vi "Finish.vi"(8 "error in (no error)":errorcluster, 11 "System Actor in":refnum<class "System Actor.lvclass">) -> (0 "error out":errorcluster, 3 "System Actor out":refnum<class "System Actor.lvclass">)   [LabVIEW 2014, in "Robot Actor Framework.lvlib" / "System Actor.lvlib" / "System Actor.lvclass"]
uses:
  System Actor.lvclass
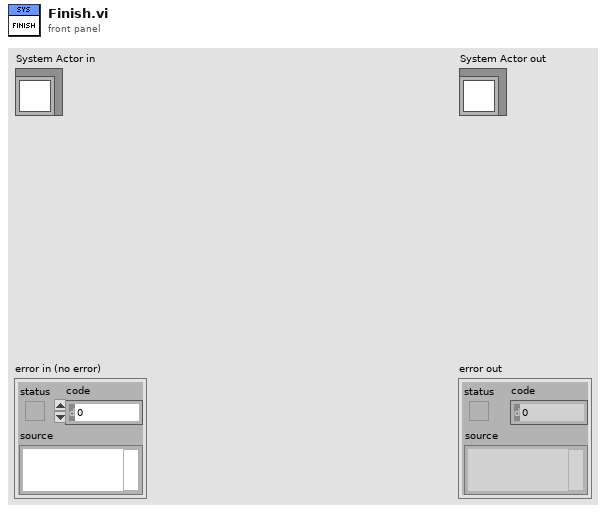
[diagram p1: front panel]
types:
  T1 = enum16{"Critical", "Error", "Warning", "Informational", "Debug"}
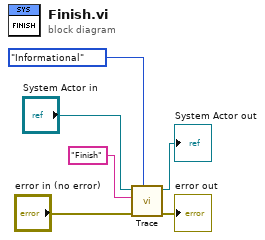
[diagram p0: block diagram]
diagram:
  n1 = call-dynamic "Trace.vi"("Trace Level"=T1."Informational", "error in (no error)"="error in (no error)", "System Action"="Finish" ("Trace Message"), "System Actor in"="System Actor in") -> ("error out"=→"error out":errorcluster, "System Actor out"=→"System Actor out":refnum<class "System Actor.lvclass">)  [unwired: 6 in]
